vi "处理文件路径.vi"(8 "错误输入":errorcluster, 11 "TDMS Files Path":path) -> (0 "错误输出":errorcluster, 1 "可用":bool, 2 "文件个数":i32, 3 "文件数组":path[](array[path]))   [LabVIEW 2018]
uses:
  <vilib>/regexp/Match Regular Expression.xnode
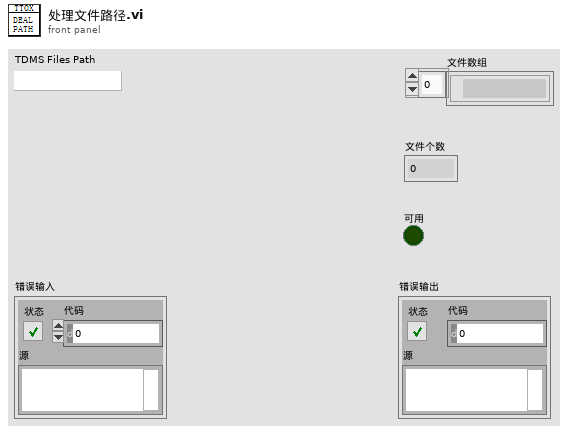
[diagram p1: front panel]
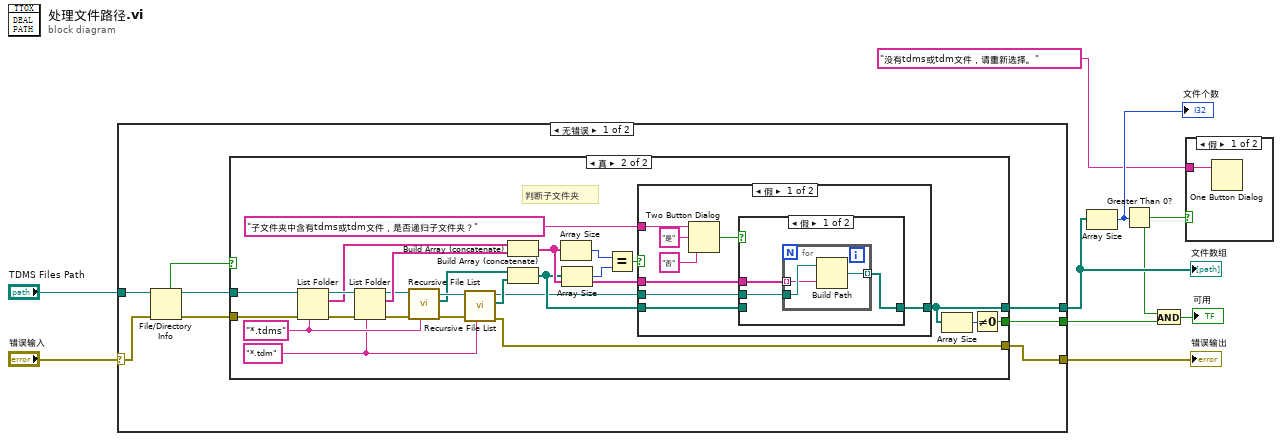
[diagram p0: block diagram]
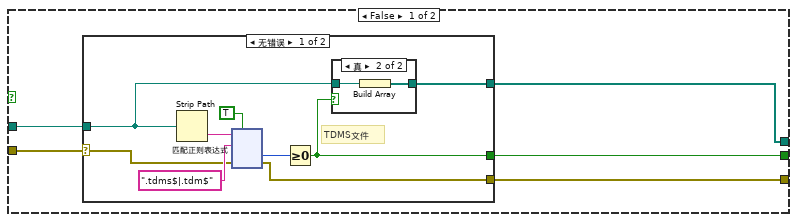
[diagram p3: hidden frame]
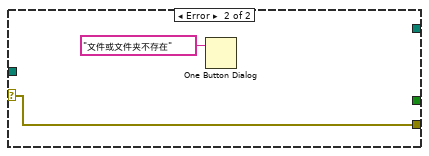
[diagram p5: hidden frame]
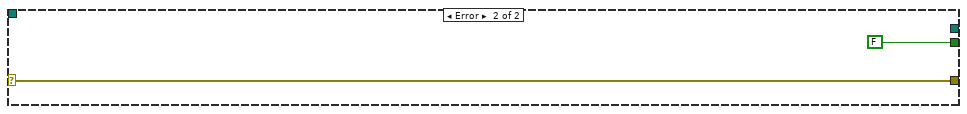
[diagram p8: hidden frame]
diagram:
  n1 = case shown="无错误" "错误输入" {
    selector: "错误输入" -> [w16 w192]
    tunnel: "TDMS Files Path" -> [w17 _]
    tunnel: [w12 FALSE] -> w3
    tunnel: [w11 w192] -> w7
    tunnel: [w10 _] -> w6
    frame No Error {
      n2 = File/Directory Info(path=w17, error in=w16) -> (path out=w14:path, directory=w15:bool, error out=w13:errorcluster)  [unwired: 4 out]
      n3 = case shown="真" w15 {
        tunnel: w14 -> [w20 w174]
        tunnel: w13 -> [w19 w173]
        tunnel: [w22 w152] -> w12
        tunnel: [w21 w161] -> w11
        tunnel: [w18 w151] -> w10
        frame False {
          n4 = case shown="无错误" w19 {
            selector: w19 -> [w26 w148]
            tunnel: [w24 _] -> w22
            tunnel: [w27 w148] -> w21
            tunnel: w20 -> [w25 _]
            tunnel: [w23 _] -> w18
            frame No Error {
              # "TDMS文件"
              n5 = Strip Path(path=w25) -> (name=w31:string)  [unwired: 1 out]
              n6 = xnode "匹配正则表达式"("输入字符串"=w31, "正则表达式"=".tdms$|.tdm$", "错误输入"=w26, "忽略大小写？(F)"=TRUE) -> ("匹配后偏移量"=w28:i32, "错误输出"=w27:errorcluster)  [unwired: 2 in, 3 out]
              n7 = Greater Or Equal To 0?(x=w28) -> (x >= 0?=w24:bool)
              n8 = case shown="真" w24 {
                tunnel: w25 -> [_ w33]
                tunnel: [_ w32] -> w23
                frame False {
                }
                frame True {
                  n9 = Build Array(w33) -> (w32:path[])
                }
              }
            }
            frame Error {
              n10 = One Button Dialog(message="文件或文件夹不存在" ("消息")) -> ()  [unwired: 1 in, 1 out]
            }
          }
        }
        frame True {
          w160 = "*.tdm" ("类型")
          w167 = "*.tdms" ("类型")
          # "判断子文件夹"
          n11 = List Folder(path=w174, pattern=w167, error in=w173) -> (path out=w172:path, filenames=w170:string[], error out=w171:errorcluster)  [unwired: 1 in, 1 out]
          n12 = List Folder(path=w172, pattern=w160, error in=w171) -> (path out=w168:path, filenames=w169:string[], error out=w166:errorcluster)  [unwired: 1 in, 1 out]
          n13 = call <vilib>:"Recursive File List.vi"("pattern"=w167, "error in (no error)"=w166, "Folder Path"=w168) -> ("error out"=w165:errorcluster, "All Files in Dir"=w163:path[], "dup Folder Path"=w164:path)  [unwired: 4 in, 2 out]
          n14 = call <vilib>:"Recursive File List.vi"("pattern"=w160, "error in (no error)"=w165, "Folder Path"=w164) -> ("error out"=w161:errorcluster, "All Files in Dir"=w162:path[], "dup Folder Path"=w153:path)  [unwired: 4 in, 2 out]
          n15 = Build Array (concatenate)(w170, w169) -> (w157:string[])
          n16 = Build Array (concatenate)(w163, w162) -> (w155:path[])
          n17 = Array Size(array=w157) -> (size(s)=w159:i32)
          n18 = Array Size(array=w155) -> (size(s)=w154:i32)
          n19 = Equal?(x=w159, y=w154) -> (x = y?=w158:bool)
          n20 = case shown="假" w158 {
            tunnel: w157 -> [w177 _]
            tunnel: "子文件夹中含有tdms或tdm文件，是否递归子文件夹？" ("消息") -> [w182 _]
            tunnel: w155 -> [w178 w190]
            tunnel: [w176 w190] -> w151
            tunnel: w153 -> [w175 _]
            frame False {
              n21 = Two Button Dialog(message=w182, 1:"否" ("F按钮名称（“取消”）"), 2:"是" ("T按钮名称（“确定”）")) -> (T button?=w179:bool)
              n22 = case shown="假" w179 {
                tunnel: w178 -> [_ w189]
                tunnel: w177 -> [w184 _]
                tunnel: [w183 w189] -> w176
                tunnel: w175 -> [w185 _]
                frame False {
                  n23 = for {
                    tunnel: w185 -> [w188]
                    tunnel: w184 -> [w187] mode=indexing
                    tunnel: [w186] -> w183 mode=indexing
                    n24 = Build Path(base path=w188, name or relative path=w187) -> (appended path=w186:path)
                  }
                }
                frame True {
                }
              }
            }
            frame True {
            }
          }
          n25 = Array Size(array=w151) -> (size(s)=w150:i32)
          n26 = Not Equal To 0?(x=w150) -> (x != 0?=w152:bool)
        }
      }
    }
    frame Error {
    }
  }
  "错误输出" <- w7
  "文件数组" <- w6
  n27 = Array Size(array=w6) -> (size(s)=w5:i32)
  "文件个数" <- w5
  n28 = Greater Than 0?(x=w5) -> (x > 0?=w2:bool)
  n29 = And(x=w2, y=w3) -> (x .and. y?=→"可用":bool)
  n30 = case shown="假" w2 {
    tunnel: "没有tdms或tdm文件，请重新选择。" -> [w193 _]
    frame False {
      n31 = One Button Dialog(message=w193) -> ()  [unwired: 1 in, 1 out]
    }
    frame True {
    }
  }
